vi "Trap Density_VT.vi"(1 "VT":dbl format="%#_4e", 2 "Dielectric":dbl format="%#_4e") -> (0 "Trap Density-VT":dbl format="%#_4e")   [LabVIEW 2012]
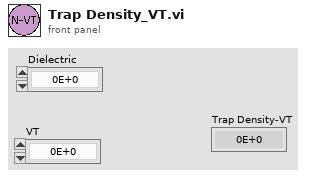
[diagram p1: front panel]
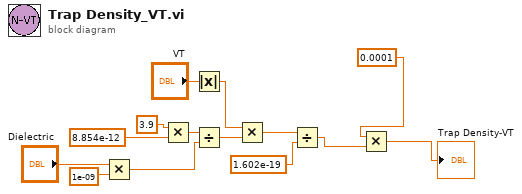
[diagram p0: block diagram]
diagram:
  n1 = Multiply(x="Dielectric", y=1e-09) -> (x*y=w11:dbl)
  n2 = Multiply(x=3.9, y=8.854e-12) -> (x*y=w9:dbl)
  n3 = Absolute Value(x="VT") -> (abs(x)=w14:dbl)
  n4 = Divide(x=w9, y=w11) -> (x/y=w5:dbl)
  n5 = Multiply(x=w14, y=w5) -> (x*y=w13:dbl)
  n6 = Divide(x=w13, y=1.602e-19) -> (x/y=w3:dbl)
  n7 = Multiply(x=0.0001, y=w3) -> (x*y=→"Trap Density-VT":dbl)
